vi "Absolute Time Chart-LV12.vi"() -> ()   [LabVIEW 2016]
panel:
  out "error out":errorcluster
  in  "stop":bool
  in  "Samples Per Second":dbl=15.0
  out "Waveform Chart":dbl(graph)=-0.7727644875559871
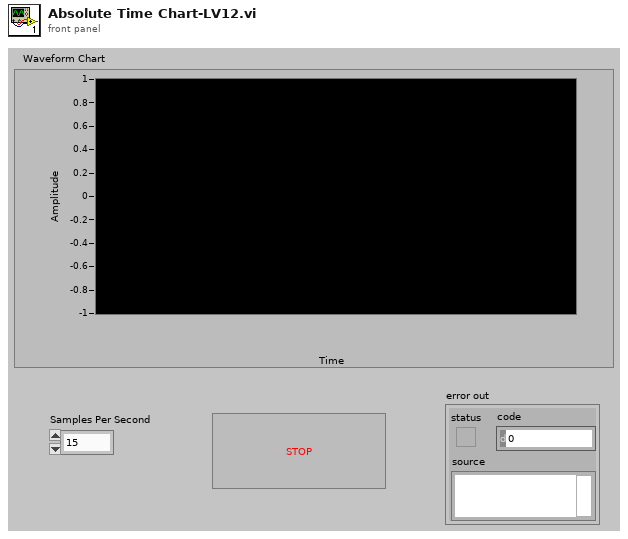
[diagram p1: front panel]
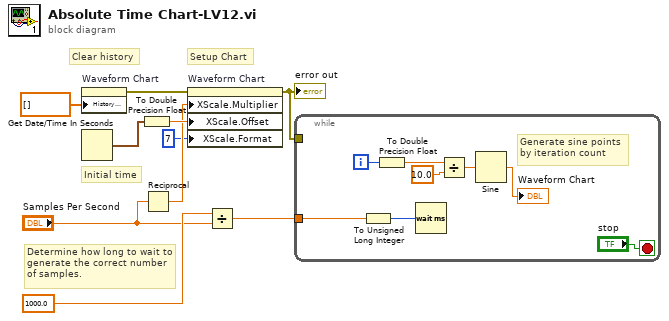
[diagram p0: block diagram]
diagram:
  # "Clear history"
  # "Initial time"
  # "Setup Chart"
  # "Determine how long to wait to generate the correct number of samples."
  n1 = property on="Waveform Chart" class="WFChart (strict)"("History Data"=dbl[] []) -> (error out=w1:errorcluster)  [unwired: 2 in, 1 out]
  n2 = Get Date/Time In Seconds() -> (seconds since 1Jan1904=w9:timestamp)
  n3 = To Double Precision Float(number=w9) -> (double precision float=w10:dbl)
  n4 = Reciprocal(x="Samples Per Second") -> (1/x=w8:dbl)
  n5 = property on="Waveform Chart" class="WFChart (strict)"(error in=w1, "XScale.Multiplier"=w8, "XScale.Offset"=w10, "XScale.Format"=u8 7 ("X Scale.Display Format:Format")) -> (error out=w6:errorcluster)  [unwired: 1 in, 1 out]
  "error out" <- w6
  n6 = Divide(x=1000.0, y="Samples Per Second") -> (x/y=w3:dbl)
  n7 = while {
    tunnel: w6 -> [_]
    tunnel: w3 -> [w14]
    i -> [w12]
    stop <- "stop" stop-if-true
    # "Generate sine points\nby iteration count"
    n8 = To Unsigned Long Integer(number=w14) -> (unsigned 32bit integer=w13:u32)
    n9 = To Double Precision Float(number=w12) -> (double precision float=w11:dbl)
    n10 = Wait (ms)(milliseconds to wait=w13) -> ()  [unwired: 1 out]
    n11 = Divide(x=w11, y=10.0) -> (x/y=w16:dbl)
    n12 = Sine(x=w16) -> (sin(x)=→"Waveform Chart":dbl)
  }
